vi "Noise-Initialize.vi"(0 "Noise":T5, 5 "Level":T3, 7 "Filter":T1 {"Stages"."IIR Filter"."Forward Coefficients" format="%.4f"; "Stages"."IIR Filter"."Reverse Coefficients" format="%.4f"}, 9 "Sampling rate (Hz)":dbl, 11 "error in (no error)":errorcluster) -> (4 "Noise Out":T5, 6 "Level Out":T3, 8 "Filter Out":T1 {"Stages"."IIR Filter"."Forward Coefficients" format="%.4f"; "Stages"."IIR Filter"."Reverse Coefficients" format="%.4f"}, 10 "Noise":dbl[](array[numeric]), 15 "error out":errorcluster)   [LabVIEW 2020]
uses:
  Controls/Advanced Filter XCtl/Filter Data.ctl
  Filter VIs/Filter-Bandwidth Units.ctl
  Noise Params.ctl
  Controls/Level XCtl/Level Data.ctl
  Controls/Level XCtl/Level Units.ctl
  Noise-Globals.vi
  Controls/Advanced Filter XCtl/Advanced Filter XCtl.xctl
  Controls/Level XCtl/Level XCtl.xctl
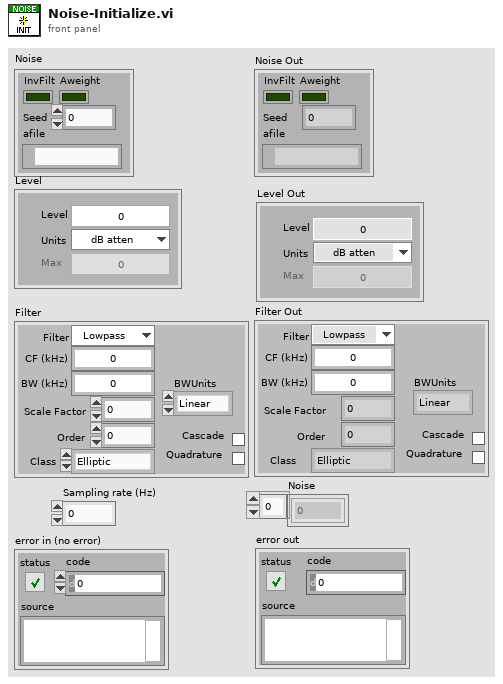
[diagram p1: front panel]
types:
  T1 = typedef "Advanced Filter XCtl.xctl/Filter Data.ctl" = cluster{"Type":enum16{"Lowpass", "Highpass", "Bandpass", "Bandstop", "OFF"}, "CF (kHz)":dbl, "BW (kHz)":dbl, "Cascade":bool, "Quadrature":bool, "Scale Factor":dbl, "Stages":cluster{"IIR Filter":cluster{"filter structure":enum32{"IIR 2nd Order", "IIR 4th Order"}, "Reverse Coefficients":dbl[], "Forward Coefficients":dbl[]}, "State":dbl[]}[], "Class":enum16{"Elliptic", "Butterworth"}, "Order":i32, "BWUnits":T2}
  T2 = typedef "Filter-Bandwidth Units.ctl" = enum16{"Linear", "Octaves", "Min-Max"}
  T3 = typedef "Level XCtl.xctl/Level Data.ctl" = cluster{"Level":dbl, "Units":T4, "Max":dbl, "Multiplier":dbl, "Cal File":path, "Cal":cluster{"Freq (Hz)":dbl[], "Mag (dB SPL)":dbl[], "Phase (deg)":dbl[]}}
  T4 = typedef "Level Units.ctl" = enum16{"dB atten", "dB SPL", "dB re 1 Vrms", "dB V/Hz½", "mW", "dB HL", "Volts", "dB mW"}
  T5 = typedef "Noise Params.ctl" = cluster{"InvFilt":bool, "Noise":dbl[], "CurPt":i32, "Aweight":bool, "Seed":i32, "afile":path}
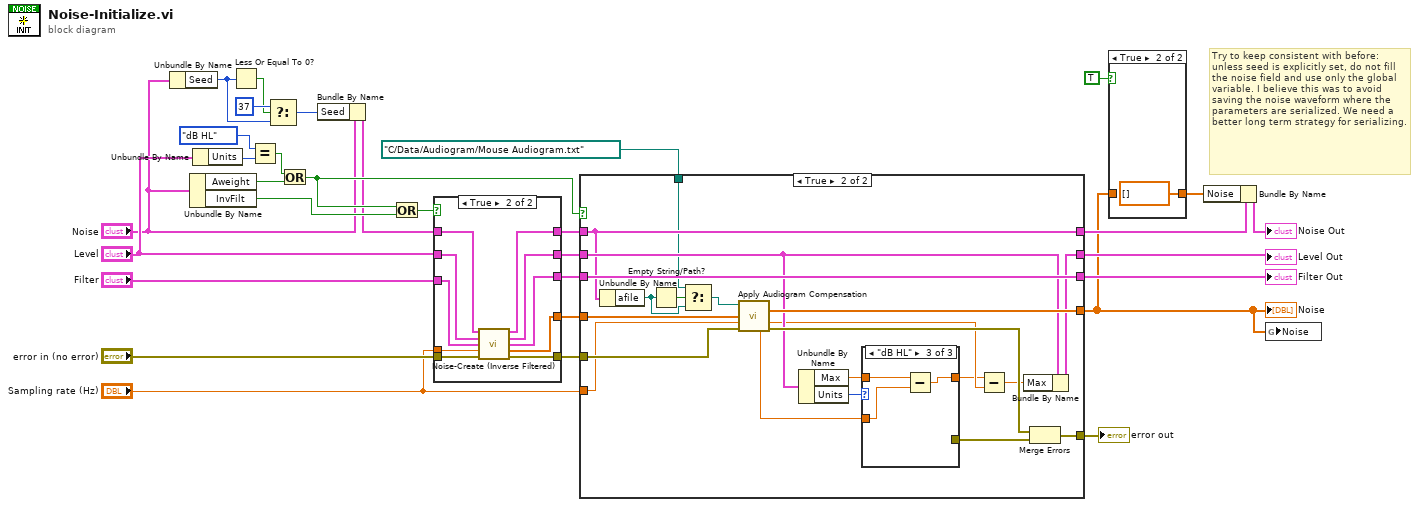
[diagram p0: block diagram]
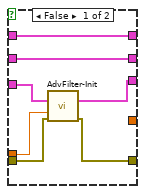
[diagram p3: hidden frame]
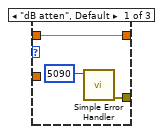
[diagram p5: hidden frame]
diagram:
  # "Try to keep consistent with before: unless seed is explicitly set, do not fill the noise field and use only the global variable. I believe this was to avoid saving the noise waveform where the parameters are serialized. We need a better long term strategy for serializing."
  n1 = Unbundle By Name("Noise") -> ("Seed"=w9:i32)
  n2 = Unbundle By Name("Noise") -> ("Aweight"=w23:bool, "InvFilt"=w31:bool)
  n3 = Unbundle By Name("Level") -> ("Units"=w14:T4)
  n4 = Less Or Equal To 0?(x=w9) -> (x <= 0?=w5:bool)
  n5 = Equal?(x=Level_Units."dB HL", y=w14) -> (x = y?=w12:bool)
  n6 = Select(t=37, s=w5, f=w9) -> (s? t:f=w7:i32)
  n7 = Or(x=w12, y=w23) -> (x .or. y?=w15:bool)
  n8 = Bundle By Name(cluster="Noise", "Seed"=w7) -> (w10:T5)
  n9 = Or(x=w15, y=w31) -> (x .or. y?=w24:bool)
  n10 = case shown="True" w24 {
    tunnel: "Sampling rate (Hz)" -> [w38 w46]
    tunnel: "error in (no error)" -> [w37 w48]
    tunnel: [w32 w42] -> w28
    tunnel: [w36 w47] -> w26
    tunnel: "Filter" -> [w35 w45]
    tunnel: w10 -> [w32 w43]
    tunnel: "Level" -> [w34 w44]
    tunnel: [w34 w41] -> w22
    tunnel: [w33 w40] -> w21
    tunnel: [_ w39] -> w20
    frame False {
      n11 = call "AdvFilter-Init.vi"("Filter"=w35, "Sampling rate (Hz)"=w38, "error in (no error)"=w37) -> ("Filter out"=w33:T1, "error out"=w36:errorcluster)  [unwired: 11 in]
    }
    frame True {
      n12 = call "Noise-Create (Inverse Filtered).vi"("Noise In"=w43, "Level In"=w44, "Filter In"=w45, "Fs (Hz)"=w46, "error in (no error)"=w48) -> ("Noise Out"=w42:T5, "Level Out"=w41:T3, "Filter Out"=w40:T1, "InvFilter Noise"=w39:dbl[], "error out"=w47:errorcluster)  [unwired: 6 in]
    }
  }
  n13 = case shown="True" w15 {
    tunnel: w28 -> [w53 w58]
    tunnel: [w53 w58] -> w19
    tunnel: [w52 w59] -> w27
    tunnel: w26 -> [w52 w73]
    tunnel: "Sampling rate (Hz)" -> [_ w72]
    tunnel: w22 -> [w51 w68]
    tunnel: w21 -> [w50 w71]
    tunnel: [w51 w66] -> w18
    tunnel: [w50 w71] -> w17
    tunnel: w20 -> [w49 w70]
    tunnel: [w49 w69] -> w4
    tunnel: path "C:/Data/Audiogram/Mouse Audiogram.txt" ("Audiogram File") -> [_ w54]
    frame False {
    }
    frame True {
      n14 = Unbundle By Name(w58) -> ("afile"=w56:path)
      n15 = Empty String/Path?(string/path=w56) -> (empty?=w57:bool)
      n16 = Select(t=w54, s=w57, f=w56) -> (s? t:f=w55:path)
      n17 = call "Apply Audiogram Compensation.vi"("Audiogram File"=w55, "Noise In"=w70, "Sampling Rate (Hz)"=w72, "error in (no error)"=w73) -> ("Compensated Noise"=w69:dbl[], "Ref Adjust"=w67:dbl, "audiogram min (dB SPL)"=w61:dbl, "error out"=w74:errorcluster)  [unwired: 8 in]
      n18 = Unbundle By Name(w68) -> ("Max"=w63:dbl, "Units"=w64:T4)
      n19 = case shown="\"dB HL\"" w64 {
        tunnel: w63 -> [w77 w78 w81]
        tunnel: [w77 w78 w80] -> w62
        tunnel: w61 -> [_ _ w79]
        tunnel: [w75 _ _] -> w60
        frame "dB atten", Default {
          n20 = call <vilib>:"Simple Error Handler.vi"("error code (no error:0)"=5090) -> ("error out"=w75:errorcluster)  [unwired: 4 in, 4 out]
        }
        frame "dB SPL" {
        }
        frame "dB HL" {
          n21 = Subtract(x=w81, y=w79) -> (x-y=w80:dbl)
        }
      }
      n22 = Subtract(x=w62, y=w67) -> (x-y=w65:dbl)
      n23 = Bundle By Name(cluster=w68, "Max"=w65) -> (w66:T3)
      n24 = Merge Errors(w74, w60) -> (w59:errorcluster)
    }
  }
  "error out" <- w27
  "Level Out" <- w18
  "Filter Out" <- w17
  "Noise" <- w4
  n25 = case shown="True" TRUE {
    tunnel: w4 -> [w82 _]
    tunnel: [w82 dbl[] [] ("Compensated Noise")] -> w3
    frame False {
    }
    frame True {
    }
  }
  n26 = Bundle By Name(cluster=w19, "Noise"=w3) -> (→"Noise Out":T5)
  n27 = global write "Noise-Globals.vi" "Noise"(w4) -> ()
